vi "subviexample.vi"() -> ()   [LabVIEW 2024]
panel:
  out "nPr":dbl
  out "nCr":dbl
  in  "r":dbl
  in  "n":dbl
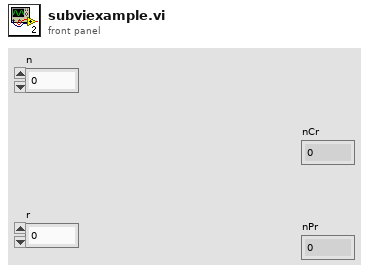
[diagram p1: front panel]
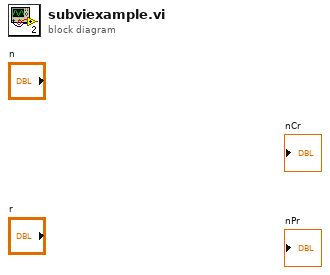
[diagram p0: block diagram]
diagram:
